vi "FailureDescription.vi"(8 "error in (no error)":errorcluster, 10 "Actual":variant, 11 "ErrorCode in":refnum<class "ErrorCode.lvclass">) -> (0 "error out":errorcluster, 2 "Failure Description":string, 3 "ErrorCode out":refnum<class "ErrorCode.lvclass">)   [LabVIEW 2017, in "Transparent Assertions.lvlib" / "ErrorCode.lvclass"]
doc: "Return the second part of the scentence \"Failed asserting that ...\""
uses:
  ErrorCode.lvclass
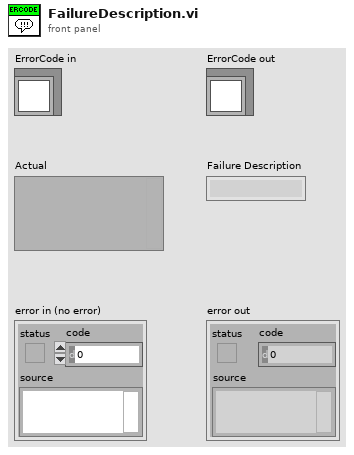
[diagram p1: front panel]
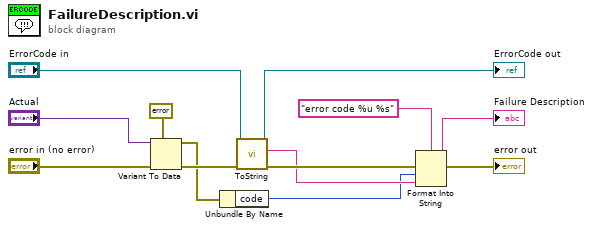
[diagram p0: block diagram]
diagram:
  n1 = Variant To Data(error in="error in (no error)", type=errorcluster {"status"=FALSE, "code"=0, "source"=""} ("error constant"), Variant="Actual") -> (data=w9:errorcluster, error out=w12:errorcluster)
  n2 = Unbundle By Name(w9) -> ("code"=w2:i32)
  n3 = call-dynamic "ToString.vi"("error in (no error)"=w12, "ErrorCode in"="ErrorCode in") -> ("error out"=w8:errorcluster, "String"=w3:string, "ErrorCode out"=→"ErrorCode out":refnum<class "ErrorCode.lvclass">)  [unwired: 7 in]
  n4 = Format Into String(format string="error code %u %s", error in=w8, w2, w3) -> (resulting string=→"Failure Description":string, error out=→"error out":errorcluster)  [unwired: 1 in]
